vi "GetControlReferences.vi"(8 "error in (no error)":errorcluster, 11 "UI_Interaction_Manager in":refnum<class "UI_Interaction_Manager.lvclass">) -> (0 "error out":errorcluster, 2 "Controls[] out":refnum<vi>[](array[refnum]), 3 "UI_Interaction_Manager out":refnum<class "UI_Interaction_Manager.lvclass">)   [LabVIEW 2011, in "UI_Interaction_Manager.lvclass"]
uses:
  UI_Interaction_Manager.lvclass
  UI_Interaction_Manager.lvclass/UI_Interaction_Manager.ctl
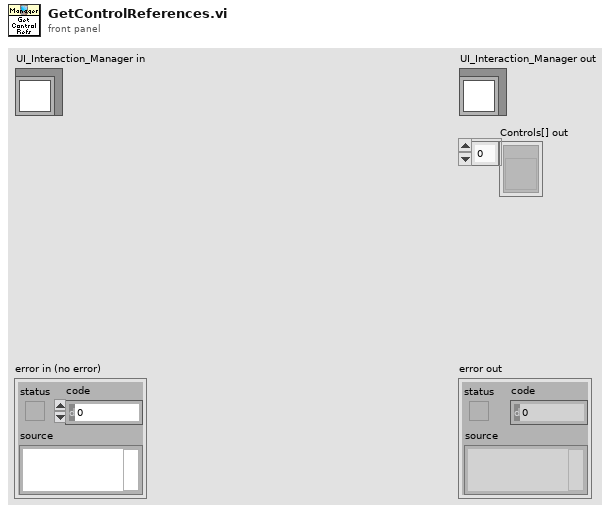
[diagram p1: front panel]
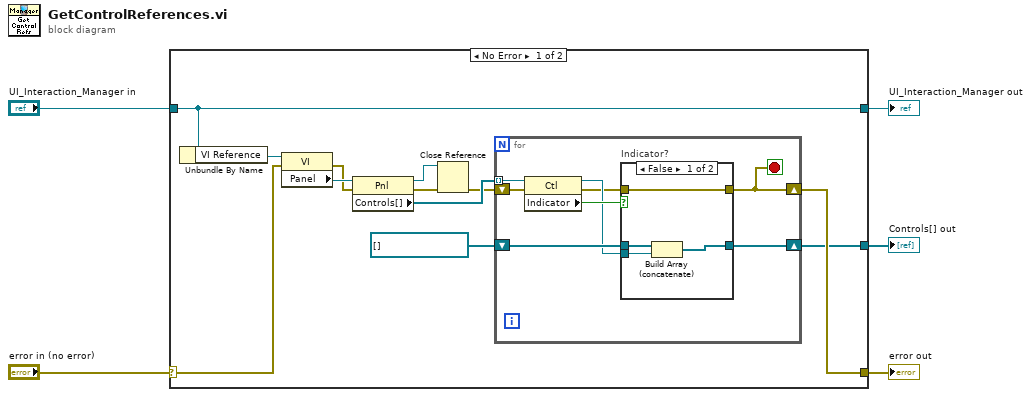
[diagram p0: block diagram]
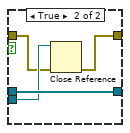
[diagram p2: hidden frame]
diagram:
  n1 = case shown="No Error" "error in (no error)" {
    selector: "error in (no error)" -> [w11 w35]
    tunnel: [w16 w35] -> w4
    tunnel: [w14 w34] -> w2
    tunnel: "UI_Interaction_Manager in" -> [w14 w34]
    tunnel: [w15 _] -> w1
    frame No Error {
      n2 = Unbundle By Name(w14) -> ("VI Reference"=w13:refnum<vi>)
      n3 = property class="VI"(reference=w13, error in=w11) -> (error out=w6:errorcluster, "Panel"=w12:refnum<vi>)  [unwired: 1 out]
      n4 = property class="Pnl"(reference=w12, error in=w6) -> (reference out=w8:refnum<vi>, error out=w9:errorcluster, "Controls[]"=w10:refnum<vi>[])
      n5 = Close Reference(reference=w8, error in (no error)=w9) -> (error out=w7:errorcluster)
      n6 = for {
        shift-right: [w23] -> w15
        shift-left: refnum<vi>[] [] -> [w24]
        shift-right: [w18] -> w16
        shift-left: w7 -> [w25]
        tunnel: w10 -> [w20] mode=indexing
        stop <- w18 stop-if-true
        n7 = property class="Ctl"(reference=w20, error in=w25) -> (reference out=w21:refnum<vi>, error out=w19:errorcluster, "Indicator"=w22:bool)
        n8 = case "Indicator?" shown="False" w22 {
          tunnel: w24 -> [w29 w33]
          tunnel: [w28 w33] -> w23
          tunnel: w21 -> [w27 w32]
          tunnel: w19 -> [w26 w31]
          tunnel: [w26 w30] -> w18
          frame False {
            n9 = Build Array (concatenate)(w29, w27) -> (w28:refnum<vi>[])
          }
          frame True {
            n10 = Close Reference(reference=w32, error in (no error)=w31) -> (error out=w30:errorcluster)
          }
        }
      }
    }
    frame Error {
    }
  }
  "error out" <- w4
  "UI_Interaction_Manager out" <- w2
  "Controls[] out" <- w1
